vi "Cross Correlation.vi"(0 "reference in":refnum<class "SigMath.lvclass">, 5 "error in (no error)":errorcluster, 6 "Weighting":u16(ring) items=["biased (N)", "unbiased (N-k)"], 7 "Sub Signals A":i32 caption="Set A", 9 "Sub Signals B":i32 caption="Set B") -> (11 "Delay (msec)":dbl, 13 "correlogram":cluster{"Ramp Pattern":dbl[], "Rxy":dbl[]}(graph), 14 "reference out":refnum<class "SigMath.lvclass">, 17 "Fs":dbl, 18 "Max Amp":dbl, 19 "error out":errorcluster)   [LabVIEW 2022 SP3, in "SigMath.lvclass"]
uses:
  SigMath.lvclass
  <vilib>/addons/Time Series Analysis/Correlation and Spectral Analysis.llb/TSA Cross-Correlation Function (Waveform).vi
  API/GSwFormDSP_class/GSwFormDSP.lvclass
  <vilib>/addons/_Advanced Signal Processing/NI_AdvSigProcTSA.lvlib
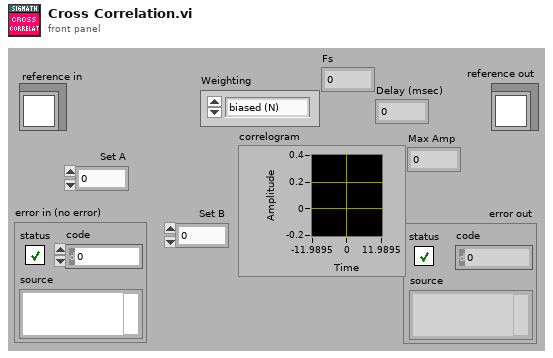
[diagram p1: front panel]
types:
  T1 = typedef "SigMath.lvclass/ObjectAttributes.ctl" = cluster{"SigMath Data":T2, "User CTRL Refs":T3}
  T2 = typedef "SigMath.lvclass/SigMath Data.ctl" = cluster{"New Time Data Obj?":bool, "GSwFormDSP":refnum<class "GSwFormDSP.lvclass">}
  T3 = typedef "SigMath.lvclass/SigMath User CTRL Refs.ctl" = cluster{"wForms":refnum<vi>, "Results wForms":refnum<vi>}
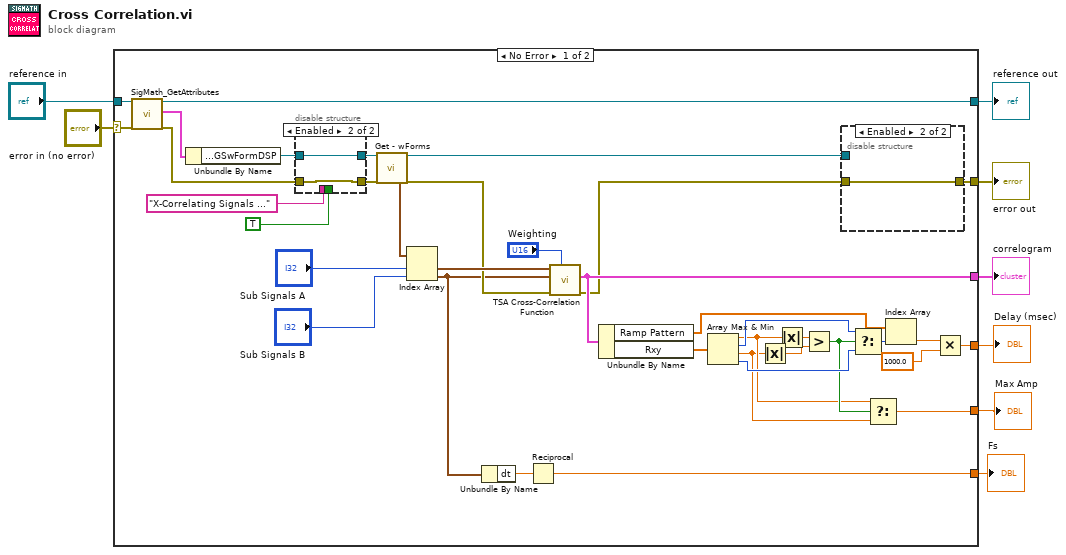
[diagram p0: block diagram]
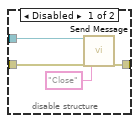
[diagram p2: hidden frame]
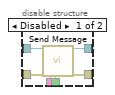
[diagram p3: hidden frame]
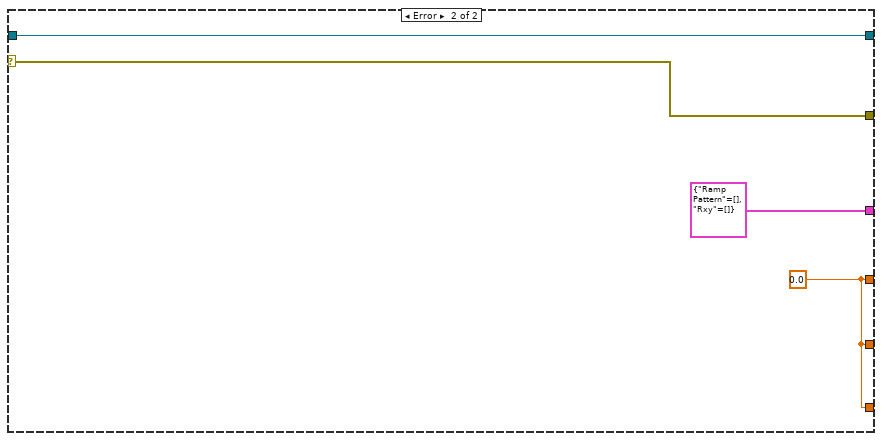
[diagram p4: hidden frame]
diagram:
  n1 = case shown="No Error" "error in (no error)" {
    selector: "error in (no error)" -> [w45 w62]
    tunnel: [w13 w62] -> w7
    tunnel: [w44 w61] -> w5
    tunnel: "reference in" -> [w43 w61]
    tunnel: [w35 cluster{"Ramp Pattern":dbl[], "Rxy":dbl[]} {"Ramp Pattern"=[], "Rxy"=[]} ("correlogram")] -> w4
    tunnel: [w25 w59] -> w3
    tunnel: [w21 w59] -> w2
    tunnel: [w9 w59] -> w1
    frame No Error {
      n2 = call "SigMath_GetAttributes.vi"("reference in"=w43, "error in (no error)"=w45) -> ("reference out"=w44:refnum<class "SigMath.lvclass">, "attributes"=w42:T1, "error out"=w15:errorcluster)  [unwired: 14 in, 1 out]
      n3 = Unbundle By Name(w42) -> ("SigMath Data.GSwFormDSP"=w18:refnum<class "GSwFormDSP.lvclass">)
      n4 = disable-structure shown="Enabled" {
        disable-tunnel: "X-Correlating Signals ..." ("Message (\"\" closes the window)") -> [w56 _]
        disable-tunnel: TRUE ("Make Cursor Busy?") -> [w55 _]
        disable-tunnel: w18 -> [w54 w58]
        disable-tunnel: [w53 w58] -> w17
        disable-tunnel: [w52 w57] -> w16
        disable-tunnel: w15 -> [w51 w57]
        frame Disabled {
          n5 = call-dynamic "Send Message.vi"("reference in"=w54, "error in (no error)"=w51, "Message (\"\" closes the window)"=w56, "Make Cursor Busy?"=w55) -> ("reference out"=w53:refnum<class "GSwFormDSP.lvclass">, "error out"=w52:errorcluster)  [unwired: 14 in]
        }
        frame Enabled {
        }
      }
      n6 = call-dynamic "Get - wForms.vi"("reference in"=w17, "error in (no error)"=w16) -> ("wForms"=w41:waveform(dbl)[], "reference out"=w12:refnum<class "GSwFormDSP.lvclass">, "error out"=w37:errorcluster)  [unwired: 14 in, 1 out]
      n7 = Index Array(array=w41, index #1="Sub Signals A", index #2="Sub Signals B") -> (element #1=w38:waveform(dbl), element #2=w11:waveform(dbl))
      n8 = Unbundle By Name(w11) -> ("dt"=w10:dbl)
      n9 = Reciprocal(x=w10) -> (1/x=w9:dbl)
      n10 = call-poly <vilib>:"TSA Cross-Correlation Function.vi"("weighting"="Weighting", "error in (no error)"=w37, "Yt"=w11, "Xt"=w38) -> ("error out"=w14:errorcluster, "correlogram"=w35:cluster{"Ramp Pattern":dbl[], "Rxy":dbl[]})  [unwired: 1 in, 5 out]
      n11 = Unbundle By Name(w35) -> ("Ramp Pattern"=w28:dbl[], "Rxy"=w34:dbl[])
      n12 = Array Max & Min(array=w34) -> (max value=w23:dbl, max index (indices)=w31:i32, min value=w22:dbl, min index (indices)=w30:i32)
      n13 = Absolute Value(x=w22) -> (abs(x)=w32:dbl)
      n14 = Absolute Value(x=w23) -> (abs(x)=w33:dbl)
      n15 = Greater?(x=w33, y=w32) -> (0:w24:bool)
      n16 = disable-structure shown="Enabled" {
        disable-tunnel: w14 -> [w48 w50]
        disable-tunnel: [w47 w50] -> w13
        disable-tunnel: w12 -> [w46 _]
        frame Disabled {
          n17 = call-dynamic "Send Message.vi"("reference in"=w46, "error in (no error)"=w48, "Message (\"\" closes the window)"="Close" ("Message (\"\" closes the window)")) -> ("error out"=w47:errorcluster)  [unwired: 15 in, 1 out]
        }
        frame Enabled {
        }
      }
      n18 = Select(t=w31, s=w24, f=w30) -> (s? t:f=w29:i32)
      n19 = Select(t=w23, s=w24, f=w22) -> (s? t:f=w21:dbl)
      n20 = Index Array(array=w28, index=w29) -> (element=w27:dbl)
      n21 = Multiply(x=w27, y=1000.0) -> (x*y=w25:dbl)
    }
    frame Error {
      w59 = 0.0
    }
  }
  "error out" <- w7
  "reference out" <- w5
  "correlogram" <- w4
  "Delay (msec)" <- w3
  "Max Amp" <- w2
  "Fs" <- w1
